vi "test.vi"() -> ()   [LabVIEW 2015]
uses:
  <vilib>/Utility/file.llb/Read Delimited Spreadsheet (DBL).vi
panel:
  out "- pin":dbl[](array[numeric])=[25.0, 11.0, 22.0, 8.0, 2.0, 16.0, 5.0, 19.0]
  out "+ pin":dbl[](array[numeric])=[12.0, 23.0, 9.0, 20.0, 14.0, 3.0, 17.0, 6.0]
  out "TTL pin":i32[](array[numeric])=[13, 24, 10, 21, 15, 4, 18, 7]
  out "mode":string[](array[string])
  out "amplitude":dbl[](array[numeric])
  out "Frequency":dbl[](array[numeric])
  out "Channel":dbl[](array[numeric])
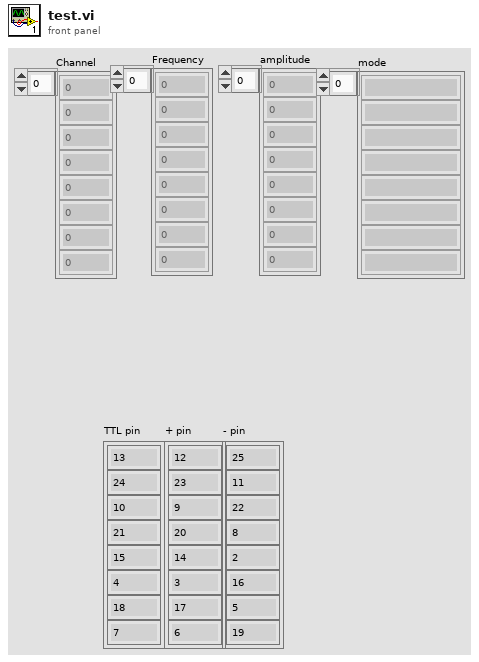
[diagram p1: front panel]
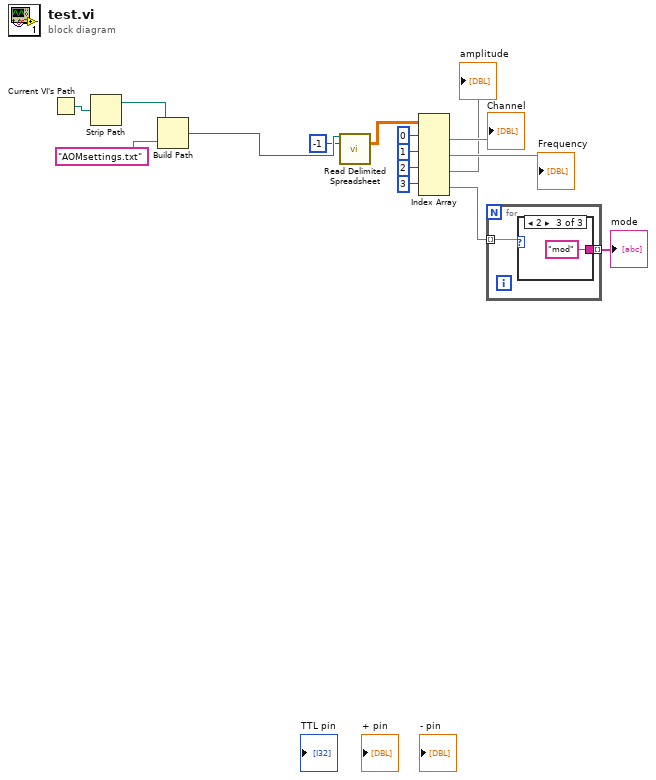
[diagram p0: block diagram]
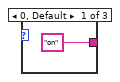
[diagram p2: hidden frame]
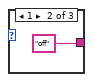
[diagram p3: hidden frame]
diagram:
  n1 = Current VI's Path() -> (path=w15:path)
  n2 = Strip Path(path=w15) -> (stripped path=w14:path)  [unwired: 1 out]
  n3 = Build Path(base path=w14, name or relative path="AOMsettings.txt") -> (appended path=w12:path)
  n4 = call-poly <vilib>:"Read Delimited Spreadsheet.vi"("file path (dialog if empty)"=w12, "number of rows (all:-1)"=-1) -> ("all rows"=w10:dbl[][])  [unwired: 8 in, 5 out]
  n5 = Index Array(array=w10, index (row) #1=0 ("index (row)"), index (row) #2=1 ("index (row)"), index (row) #3=2 ("index (row)"), index (row) #4=3 ("index (row)")) -> (element #1=→"Channel":dbl[], element #2=→"Frequency":dbl[], element #3=→"amplitude":dbl[], element #4=w2:dbl[])  [unwired: 4 in]
  n6 = for {
    tunnel: w2 -> [w17] mode=indexing
    tunnel: [w16] -> w1 mode=indexing
    n7 = case shown="2" w17 {
      tunnel: ["on" "off" "mod"] -> w16
      frame 0, Default {
      }
      frame 1 {
      }
      frame 2 {
      }
    }
  }
  "mode" <- w1
